vi "Get Physical Channels and Rate for DSA.vi"(11 "device name":string) -> (1 "maximum rate":dbl, 3 "physical channels":tag[](array[tag]))   [LabVIEW 2024, in "Dynamic Signal Acquisition (Interactive) UI.lvlib"]
doc: "For an input device, this VI gets the physical channels and the maximum sample rate. If the input device is empty, this VI looks through all devices on the system and returns the physical channels on the first DSA device detected. If there are no DSA devices, the physical channels for the last device are returned."
uses:
  <vilib>/Utility/error.llb/Trim Whitespace One-Sided.vi
  <vilib>/regexp/Match Regular Expression.xnode
  Dynamic Signal Acquisition (Interactive) UI.lvlib
  <resource>/objmgr/daqmx.rc
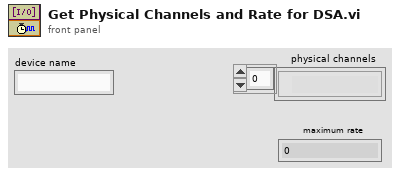
[diagram p1: front panel]
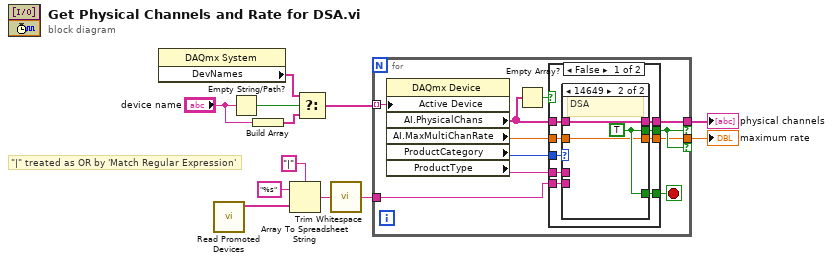
[diagram p0: block diagram]
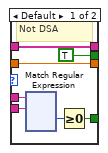
[diagram p2: hidden frame]
diagram:
  # "\"|\" treated as OR by 'Match Regular Expression'"
  n1 = property class="DAQmx System"() -> ("DevNames"=w9:tag[])  [unwired: 2 in, 2 out]
  n2 = call "Read Promoted Devices.vi"() -> ("promoted devices"=w5:string[])  [unwired: 10 in, 1 out]
  n3 = Empty String/Path?(string/path="device name") -> (empty?=w10:bool)
  n4 = Build Array("device name") -> (w8:string[])
  n5 = Array To Spreadsheet String(delimiter (Tab)="|" ("delimiter"), array=w5, 3:"%s" ("format string")) -> (spreadsheet string=w2:string)
  n6 = Select(t=w9, s=w10, f=w8) -> (s? t:f=w6:string[])
  n7 = call <vilib>:"Trim Whitespace.vi"("string"=w2) -> ("trimmed string"=w1:string)  [unwired: 1 in]
  n8 = for {
    tunnel: w6 -> [w23] mode=indexing
    tunnel: [w21] -> w11 if=w17
    tunnel: [w14] -> w12 if=w17
    tunnel: w1 -> [w13]
    stop <- w20 stop-if-true
    n9 = property class="DAQmx Device"("Active Device"=w23) -> ("AI.PhysicalChans"=w19:tag[], "AI.MaxMultiChanRate"=w15:dbl, "ProductCategory"=w18:i32, "ProductType"=w16:string)  [unwired: 2 in, 2 out]
    n10 = Empty Array?(array=w19) -> (empty?=w22:bool)
    n11 = case shown="False" w22 {
      tunnel: w18 -> [w32 _]
      tunnel: w19 -> [w31 w161]
      tunnel: [w30 w161] -> w21
      tunnel: [w29 _] -> w17
      tunnel: [w28 _] -> w20
      tunnel: w16 -> [w27 _]
      tunnel: w13 -> [w26 _]
      tunnel: [w25 w160] -> w14
      tunnel: w15 -> [w24 w160]
      frame False {
        n12 = case shown="14649" w32 {
          tunnel: w31 -> [w39 w159]
          tunnel: [w39 w159] -> w30
          tunnel: [TRUE w158] -> w29
          tunnel: [w37 w158] -> w28
          tunnel: w27 -> [w36 _]
          tunnel: w26 -> [w34 _]
          tunnel: [w33 w157] -> w25
          tunnel: w24 -> [w33 w157]
          frame Default {
            # "Not DSA"
            n13 = xnode "Match Regular Expression"("input string"=w36, "regular expression"=w34) -> ("offset past match"=w35:i32)  [unwired: 4 in, 4 out]
            n14 = Greater Or Equal To 0?(x=w35) -> (x >= 0?=w37:bool)
          }
          frame 14649 {
            w158 = TRUE
            # "DSA"
          }
        }
      }
      frame True {
      }
    }
  }
  "maximum rate" <- w12
  "physical channels" <- w11
